vi "ryTimer Set Properties.vi"(8 "error in (no error)":errorcluster, 10 "Properties":refnum<data-value>, 11 "ryTimer in":refnum<class "ryTimer.lvclass">) -> (0 "error out":errorcluster, 3 "ryTimer out":refnum<class "ryTimer.lvclass">)   [LabVIEW 2021, in "ryTimer.lvclass"]
uses:
  ryTimer.lvclass
  TypeDefs/ryTimer Properties.ctl
  ryTimer.lvclass/ryTimer.ctl
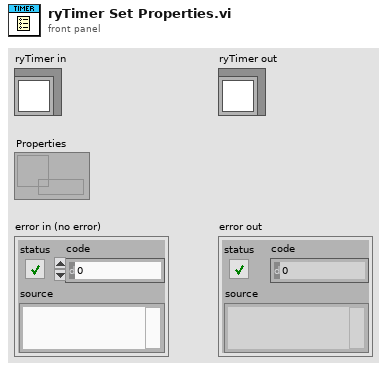
[diagram p1: front panel]
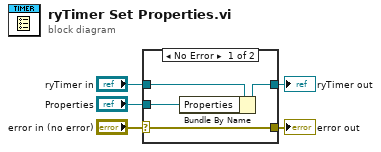
[diagram p0: block diagram]
diagram:
  n1 = case shown="No Error" "error in (no error)" {
    selector: "error in (no error)" -> [w9 w10]
    tunnel: [w9 w10] -> w4
    tunnel: [w7 w11] -> w2
    tunnel: "ryTimer in" -> [w8 w11]
    tunnel: "Properties" -> [w6 _]
    frame No Error {
      n2 = Bundle By Name(cluster=w8, "Properties"=w6) -> (w7:refnum<class "ryTimer.lvclass">)
    }
    frame Error {
    }
  }
  "error out" <- w4
  "ryTimer out" <- w2
